vi "Minusculas (2).vi"(11 "Palabra":string) -> (1 "Boolean":bool, 2 "Numeric":u8, 3 "string":string)   [LabVIEW 2020]
doc: "Darlin y Miller: Subvi que detecta letras minusculas por medio de la Tabla Ascii"
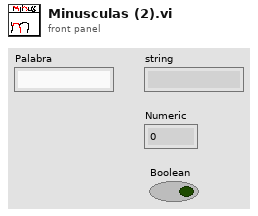
[diagram p1: front panel]
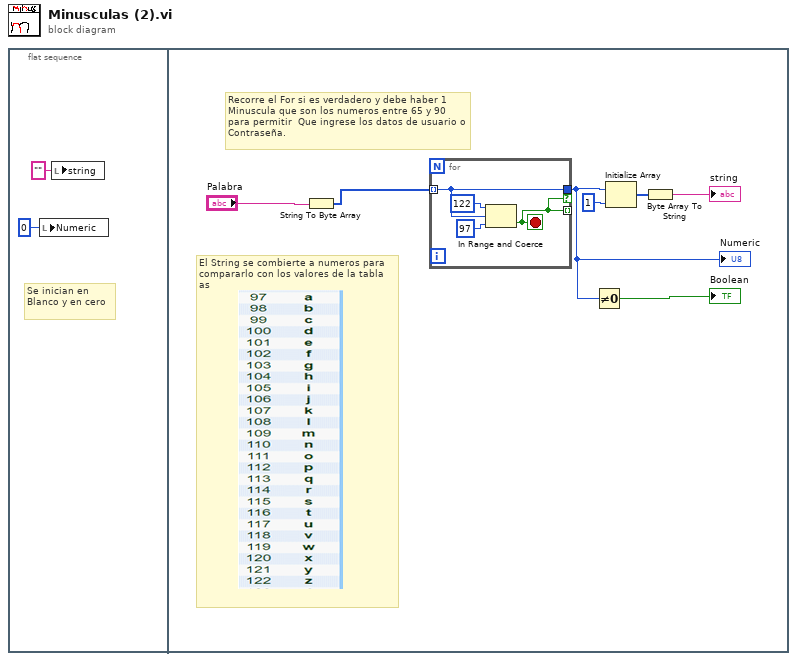
[diagram p0: block diagram]
diagram:
  n1 = flat-sequence {
    frame #0 {
      # "Se inician en Blanco y en cero"
      n2 = local write "Numeric"(u8 0 ("Numeric")) -> ()
      n3 = local write "string"("" ("string")) -> ()
    }
    frame #1 {
      # "El String se combierte a numeros para  compararlo con los valores de la tabla as"
      # "Recorre el For si es verdadero y debe haber 1 Minuscula que son los numeros entre 65 y 90 para permitir  Que ingrese los datos de usuario o Contraseña."
      n4 = String To Byte Array(string="Palabra") -> (unsigned byte array=w9:u8[])
      n5 = for {
        tunnel: w9 -> [w10] mode=indexing
        tunnel: [w10] -> w5 if=w11
        tunnel: [w11] -> _ mode=indexing
        stop <- w11 stop-if-true
        n6 = In Range and Coerce(upper limit=u8 122, x=w10, lower limit=u8 97) -> (In Range?=w11:bool)  [unwired: 1 out]
      }
      "Numeric" <- w5
      n7 = Not Equal To 0?(x=w5) -> (x != 0?=→"Boolean":bool)
      n8 = Initialize Array(w5, 1 ("dimension size")) -> (w6:u8[])
      n9 = Byte Array To String(unsigned byte array=w6) -> (string=→"string":string)
    }
  }
